vi "SaveBiasSet.vi"(0 "Application ref in":refnum<vi>, 1 "Bias (V)":sgl format="%_5p", 3 "error in (no error)":errorcluster) -> (7 "Application ref out":refnum<vi>, 10 "Error out":errorcluster)   [LabVIEW 2014]
uses:
  <userlib>/Nanonis Prog Interface V5/Nanonis Prog Interface.lvlib
panel:
  in  "Bias (V)/sec":sgl=0.01 format="%_5p"
  in  "milliseconds to wait":u32=200
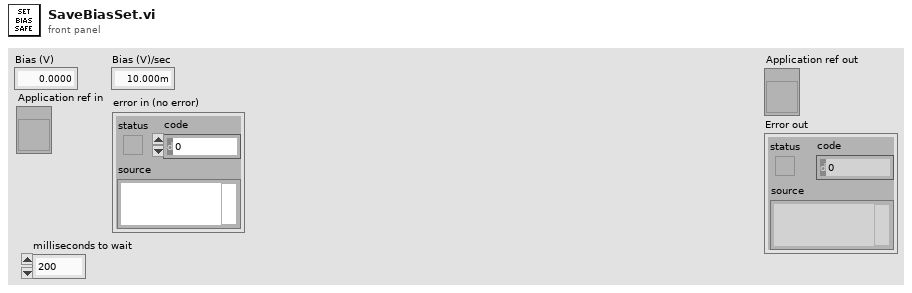
[diagram p1: front panel]
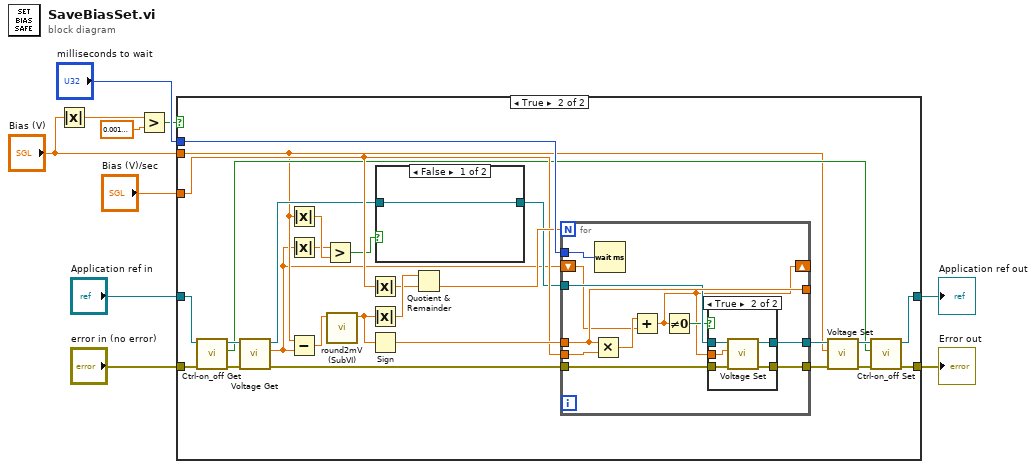
[diagram p0: block diagram]
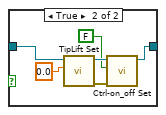
[diagram p3: hidden frame]
diagram:
  n1 = Absolute Value(x="Bias (V)") -> (abs(x)=w3:sgl)
  n2 = Greater?(x=w3, y=sgl 0.001) -> (0:w7:bool)
  n3 = case shown="True" w7 {
    tunnel: "Application ref in" -> [w12 w28]
    tunnel: "Bias (V)" -> [_ w17]
    tunnel: "error in (no error)" -> [w11 w20]
    tunnel: [w11 w21] -> w9
    tunnel: "milliseconds to wait" -> [_ w39]
    tunnel: "Bias (V)/sec" -> [_ w31]
    tunnel: [w12 w22] -> w1
    frame False {
    }
    frame True {
      n4 = call <userlib>:"Ctrl-on_off Get.vi"("error in (no error)"=w20, "Application ref in"=w28) -> ("error out"=w19:errorcluster, "Z-Controller on/off status"=w18:bool, "Application ref out"=w27:refnum<vi>)  [unwired: 7 in]
      n5 = call <userlib>:"Voltage Get.vi"("error in (no error)"=w19, "Application ref in"=w27) -> ("error out"=w38:errorcluster, "Bias (V)"=w16:sgl, "Application ref out"=w26:refnum<vi>)  [unwired: 7 in]
      n6 = Absolute Value(x=w17) -> (abs(x)=w14:sgl)
      n7 = Absolute Value(x=w16) -> (abs(x)=w13:sgl)
      n8 = Subtract(x=w17, y=w16) -> (x-y=w36:sgl)
      n9 = Greater?(x=w13, y=w14) -> (0:w15:bool)
      n10 = call "round2mV (SubVI).vi"("Numeric in"=w36) -> ("Numeric out"=w33:dbl)  [unwired: 10 in]
      n11 = Absolute Value(x=w31) -> (abs(x)=w32:sgl)
      n12 = Absolute Value(x=w33) -> (abs(x)=w34:dbl)
      n13 = Sign(1:w33) -> (0:w37:dbl)
      n14 = case shown="False" w15 {
        tunnel: w26 -> [w40 w42]
        tunnel: [w40 w41] -> w25
        frame False {
        }
        frame True {
          n15 = call <userlib>:"TipLift Set.vi"("TipLift (m)"=sgl 0.0, "Application ref in"=w42) -> ("error out"=w46:errorcluster, "Application ref out"=w45:refnum<vi>)  [unwired: 8 in]
          n16 = call <userlib>:"Ctrl-on_off Set.vi"("error in (no error)"=w46, "Z Controller ON/OFF"=FALSE, "Application ref in"=w45) -> ("Application ref out"=w41:refnum<vi>)  [unwired: 7 in, 1 out]
        }
      }
      n17 = Quotient & Remainder(x=w34, y=w32) -> (floor(x/y)=w35:dbl)  [unwired: 1 out]
      n18 = for {
        N: w35 -> [_]
        tunnel: w25 -> [w50]
        tunnel: [w57] -> w30
        tunnel: w38 -> [w51]
        tunnel: [w56] -> w29
        tunnel: w39 -> [w55]
        tunnel: w31 -> [w54]
        tunnel: w37 -> [w52]
        tunnel: [w52] -> _
        shift-right: [w47] -> _
        shift-left: w16 -> [w49]
        n19 = Multiply(x=w52, y=w54) -> (x*y=w53:dbl)
        n20 = Wait (ms)(milliseconds to wait=w55) -> ()  [unwired: 1 out]
        n21 = Add(x=w53, y=w49) -> (x+y=w47:dbl)
        n22 = Not Equal To 0?(x=w47) -> (x != 0?=w48:bool)
        n23 = case shown="True" w48 {
          tunnel: [w59 w64] -> w57
          tunnel: [w58 w63] -> w56
          tunnel: w51 -> [w58 w62]
          tunnel: w50 -> [w59 w61]
          tunnel: w47 -> [_ w60]
          frame False {
          }
          frame True {
            n24 = call <userlib>:"Voltage Set.vi"("Error in (no error)"=w62, "Bias (V)"=w60, "Application ref in"=w61) -> ("Error out"=w63:errorcluster, "Application ref out"=w64:refnum<vi>)  [unwired: 7 in]
          }
        }
      }
      n25 = call <userlib>:"Voltage Set.vi"("Error in (no error)"=w29, "Bias (V)"=w17, "Application ref in"=w30) -> ("Error out"=w23:errorcluster, "Application ref out"=w24:refnum<vi>)  [unwired: 7 in]
      n26 = call <userlib>:"Ctrl-on_off Set.vi"("error in (no error)"=w23, "Z Controller ON/OFF"=w18, "Application ref in"=w24) -> ("error out"=w21:errorcluster, "Application ref out"=w22:refnum<vi>)  [unwired: 7 in]
    }
  }
  "Application ref out" <- w1
  "Error out" <- w9
